vi "Tag-FPGA-))Channel-NoOp.vi"(8 "abort (F)":bool, 10 "element in":bool, 11 "channelOp":T1) -> (0 "aborted?":bool, 2 "element out":i32, 3 "sequence":i16)   [LabVIEW 2020, in "Tag-bool.lvlib"]
uses:
  <extravilib>/ChannelInstances/Tag-bool.lvlib
  <extravilib>/ChannelInstances/Tag-bool/ChannelOp.ctl
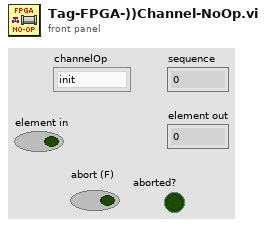
[diagram p1: front panel]
types:
  T1 = typedef "Tag-bool.lvlib/ChannelOp.ctl" = enum16{"init", "write", "read", "probe"}
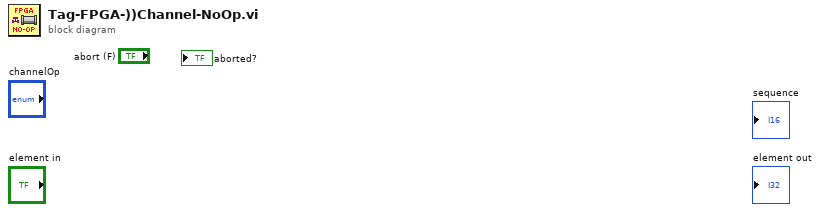
[diagram p0: block diagram]
diagram:
